vi "Main.vi"(8 "error in (no error)":errorcluster, 11 "UI in":refnum<class "UI.lvclass">) -> (0 "error out":errorcluster, 3 "UI out":refnum<class "UI.lvclass">)   [LabVIEW 2018]
uses:
  UI/UI.lvclass
  UI/UI.lvclass/UI.ctl
  UI/setEmbeddedVI.vi
panel:
  in  "Stop Button":bool
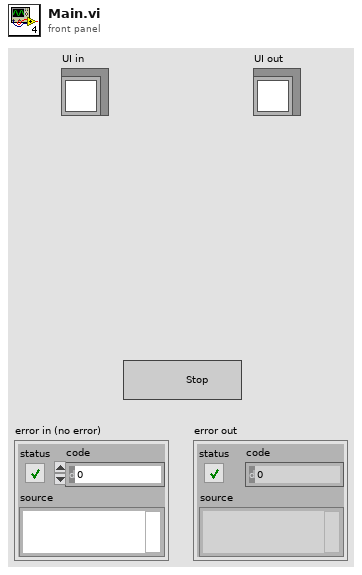
[diagram p1: front panel]
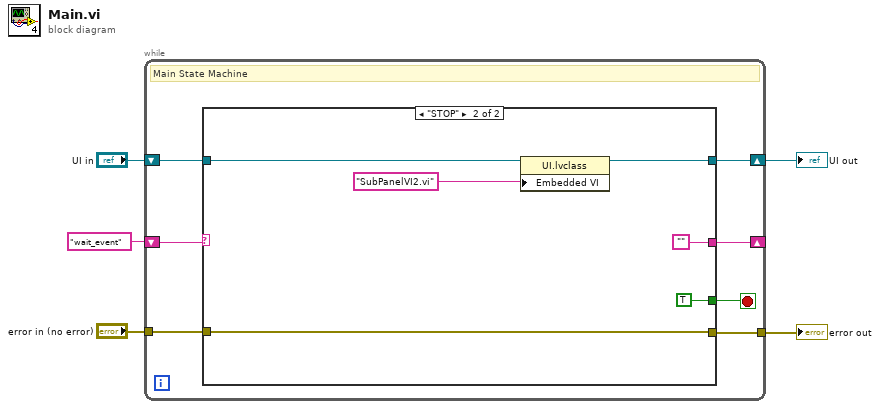
[diagram p0: block diagram]
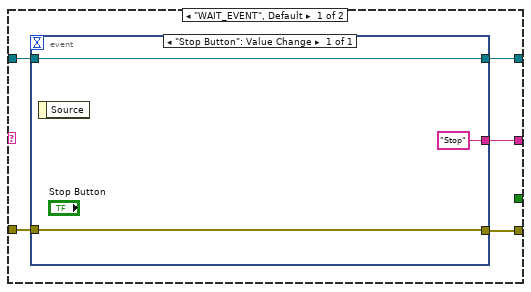
[diagram p2: hidden frame]
diagram:
  n1 = while {
    shift-right: [w11] -> w2
    shift-left: "UI in" -> [w12]
    tunnel: [w10] -> w4
    tunnel: "error in (no error)" -> [w9]
    shift-right: [w8] -> _
    shift-left: "wait_event" -> [w6]
    stop <- w7 stop-if-true
    # "Main State Machine"
    n2 = case shown="\"STOP\"" w6 {
      tunnel: w12 -> [w17 w23]
      tunnel: [w16 w24] -> w11
      tunnel: [w15 w26] -> w10
      tunnel: w9 -> [w14 w26]
      tunnel: [w13 ""] -> w8
      tunnel: [_ TRUE] -> w7
      frame "WAIT_EVENT", Default {
        n3 = event shown="[0] \"Stop Button\": Value Change" {
          selector: _ -> [_]
          dyn-events: _ -> [_]
          timeout: _ -> [_]
          tunnel: [w19] -> w16
          tunnel: w17 -> [w19]
          tunnel: [w20] -> w15
          tunnel: w14 -> [w20]
          tunnel: ["Stop"] -> w13
          event "Stop Button": Value Change {
            n4 = event-data() -> ()  [unwired: 1 in, 1 out]
          }
        }
      }
      frame "STOP" {
        n5 = property class="UI.lvclass"(reference=w23, "Embedded VI"="SubPanelVI2.vi" ("String <Replace Me>")) -> (reference out=w24:refnum<class "UI.lvclass">)  [unwired: 1 in, 1 out]
      }
    }
  }
  "UI out" <- w2
  "error out" <- w4
